vi "LVClasse_SurfaceFloat Get Dimension.vi"(0 "SurfaceFloat in":refnum<class "SurfaceFloat.lvclass">, 11 "error in (no error)":errorcluster) -> (4 "SurfaceFloat out":refnum<class "SurfaceFloat.lvclass">, 6 "Dimensions_um":T1, 15 "error out":errorcluster)   [LabVIEW 2020, in "SurfaceFloat.lvclass"]
doc: "Get Surface properties.\n\n--------------------------------------------------------------------------------\n\n<B>SurfaceIn </B> : Surface object.\n<B>SurfaceOut </B> : Surface object.\n<B>dimensions </B> : Surface dimensions (width, height).\n<B>steps </B> : Physical step x and y between the surface elements (um).\n<B>ErrorIn </B> : Error\n<B>ErrorOut </B> : Error\n\n--------------------------------------------------------------------------------"
uses:
  SurfaceFloat.lvclass
  General dimensions definition.ctl
  Point2D.ctl
  Point2Df.ctl
  SurfaceFloat.lvclass/SurfaceFloat.ctl
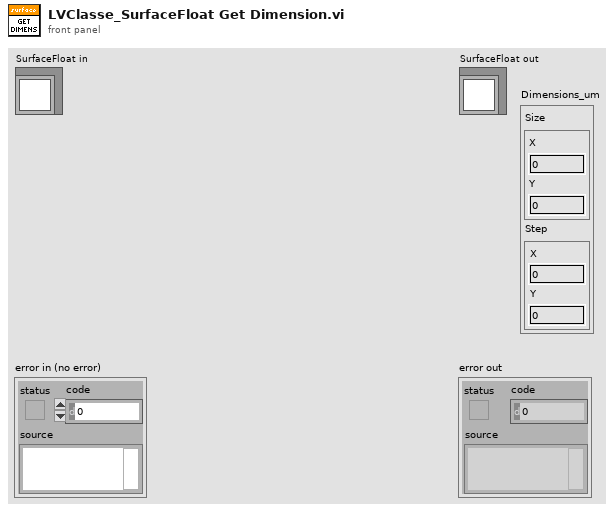
[diagram p1: front panel]
types:
  T1 = typedef "General dimensions definition.ctl" = cluster{"Size":T2, "Step":T3}
  T2 = typedef "Point2D.ctl" = cluster{"X":u32, "Y":u32}
  T3 = typedef "Point2Df.ctl" = cluster{"X":sgl, "Y":sgl}
  T4 = typedef "ClassID.ctl" = i64
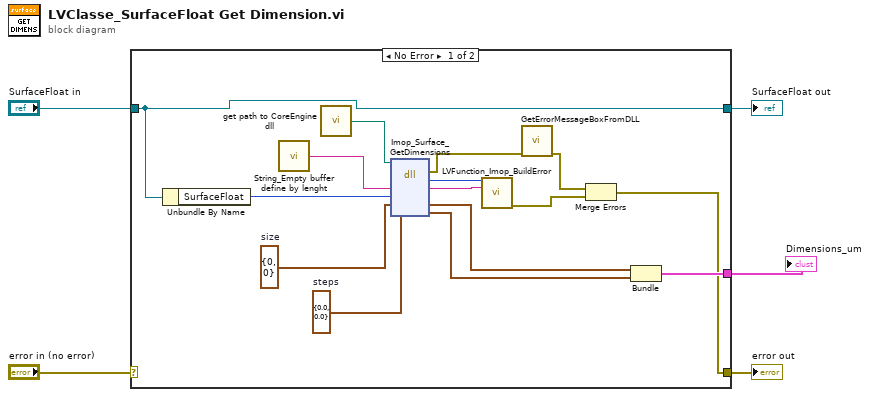
[diagram p0: block diagram]
diagram:
  n1 = case shown="No Error" "error in (no error)" {
    selector: "error in (no error)" -> [_ w22]
    tunnel: [w6 w22] -> w4
    tunnel: [w13 w21] -> w2
    tunnel: "SurfaceFloat in" -> [w13 w21]
    tunnel: [w10 _] -> w1
    frame No Error {
      w14 = T3 {"X"=0.0, "Y"=0.0}  # steps
      w15 = T2 {"X"=0, "Y"=0}  # size
      n2 = Unbundle By Name(w13) -> ("SurfaceFloat"=w12:T4)
      n3 = call "String_Empty buffer define by lenght.vi"() -> ("Empty buffer"=w18:string)  [unwired: 1 in]
      n4 = call "get path to CoreEngine dll.vi"() -> ("path to wavekit library"=w17:path)  [unwired: 14 in, 1 out]
      n5 = dll-call lib="D:/2_trunk/Soft_haso/ImOpCoreEngine4_LV2011/DLLs/ImopEngine4_vc100.dll" fn="Imop_Surface_GetDimensions"(path in=w17, "message"=w18, "surface"=w12, "size"=w15, "steps"=w14) -> (error out=w16:errorcluster, "return type"=w20:i32, "message"=w19:string, "size"=w11:T2, "steps"=w9:T3)  [unwired: 3 in, 1 out]
      n6 = call "LVFunction_Imop_BuildError.vi"("code"=w20, "String to Prepend to source (\"\")"=w19) -> ("error out"=w7:errorcluster)  [unwired: 13 in]
      n7 = call "GetErrorMessageBoxFromDLL.vi"("error IN"=w16) -> ("error OUT"=w8:errorcluster)  [unwired: 10 in]
      n8 = Merge Errors(w8, w7) -> (w6:errorcluster)
      n9 = Bundle("size"=w11, "steps"=w9) -> (w10:cluster{"size":T2, "steps":T3})  [unwired: 1 in]
    }
    frame Error {
    }
  }
  "error out" <- w4
  "SurfaceFloat out" <- w2
  "Dimensions_um" <- w1
